vi "Dvmg Get Dev Count.vi"(8 "error in (no error)":errorcluster, 11 "perc":i32) -> (0 "error out":errorcluster, 2 "function return":i32, 3 "perc out":i32)   [LabVIEW 2011, in "LVH-Adept.lvlib" / "DPCUTIL.lvlib"]
doc: "DPCAPI INT32 DvmgGetDevCount(ERC * perc);"
uses:
  DPCUTIL.lvlib
  dpcutil.dll
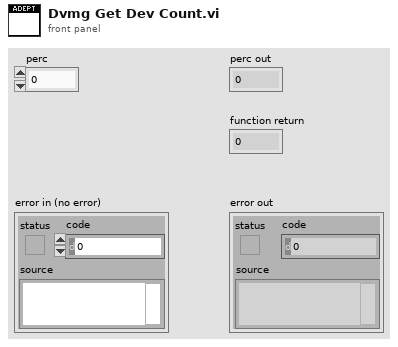
[diagram p1: front panel]
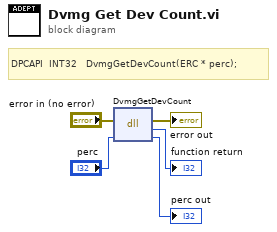
[diagram p0: block diagram]
diagram:
  # "DPCAPI  INT32   DvmgGetDevCount(ERC * perc);"
  n1 = dll-call lib="dpcutil.*" fn="DvmgGetDevCount"(error in="error in (no error)", "perc"="perc") -> (error out=→"error out":errorcluster, "return type"=→"function return":i32, "perc"=→"perc out":i32)  [unwired: 2 in, 1 out]
